vi "Controls Loop.vi"(8 "error in":errorcluster, 10 "Controls[]":refnum<vi>[](array[refnum]), 11 "Material-Scheme in":refnum<class "Material-Scheme.lvclass">) -> (0 "error out":errorcluster)   [LabVIEW 2021, in "TSC Material Theme.lvlib" / "Material-Scheme.lvclass"]
doc: "loop through all the controls on a panel in order to change the appearance\n\n<b>Code Developed By:</b>\nTechnology Service Corporation\nwww.tsc.com/atcs\n\nDeveloper:\nDaniel Coons"
uses:
  Material-Scheme.lvclass
  Material-Scheme.lvclass/Material-Scheme.ctl
  <vilib>/Utility/miscctls.llb/LVRowAndColumnTypeDef.ctl
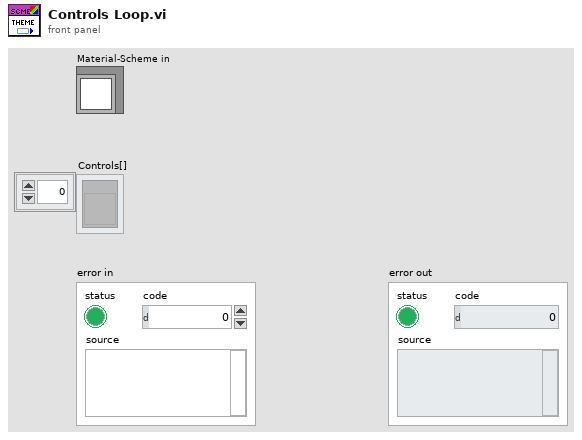
[diagram p1: front panel]
types:
  T1 = typedef "LVRowAndColumnTypeDef.ctl" = cluster{"Row":i32, "Column":i32}
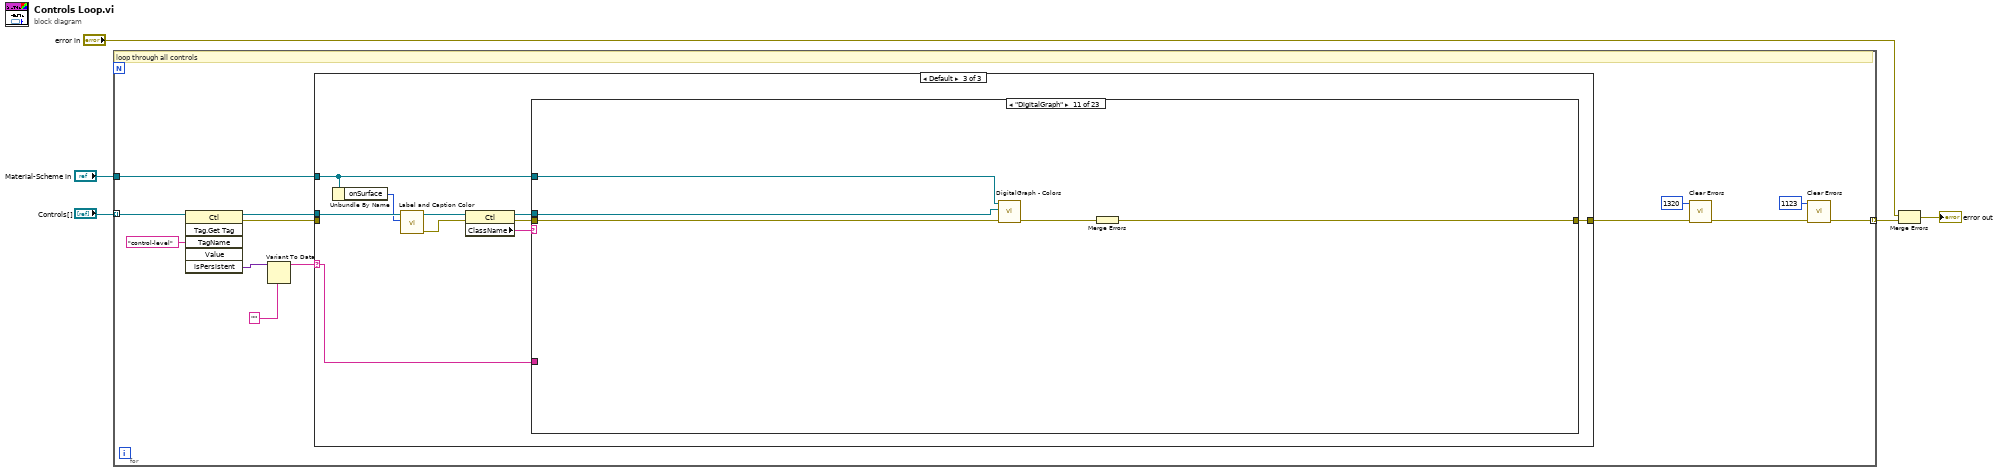
[diagram p0: block diagram]
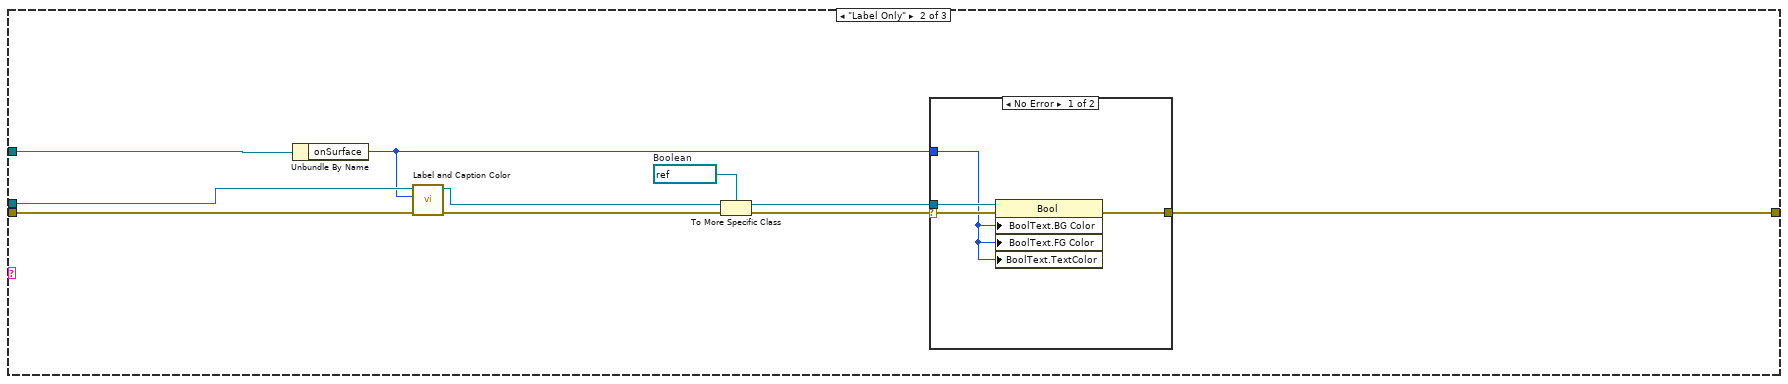
[diagram p3: hidden frame]
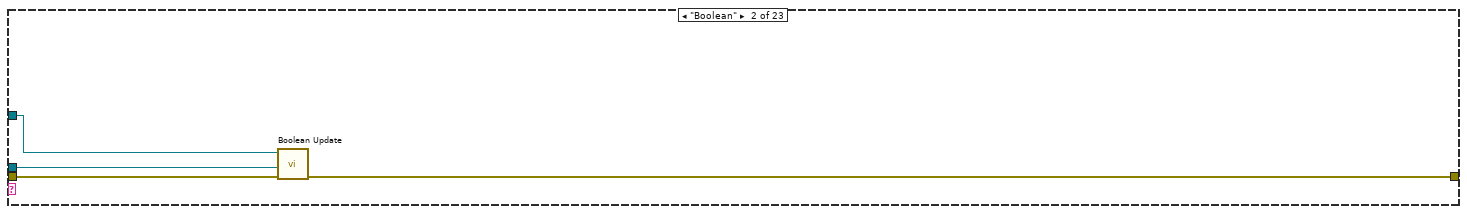
[diagram p6: hidden frame]
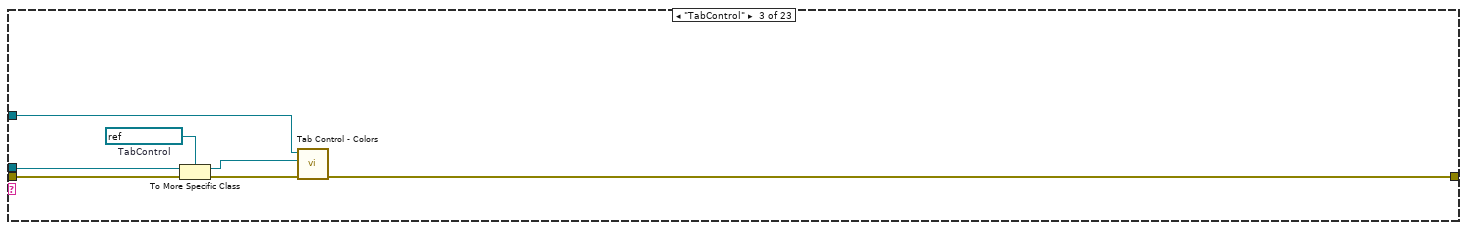
[diagram p7: hidden frame]
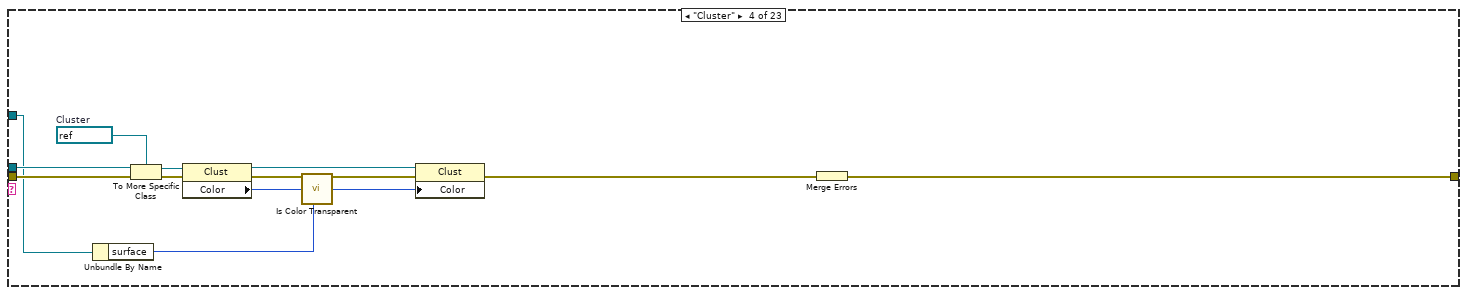
[diagram p8: hidden frame]
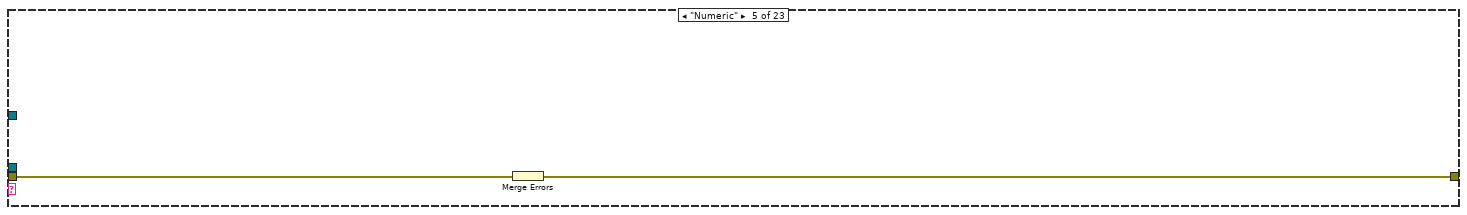
[diagram p9: hidden frame]
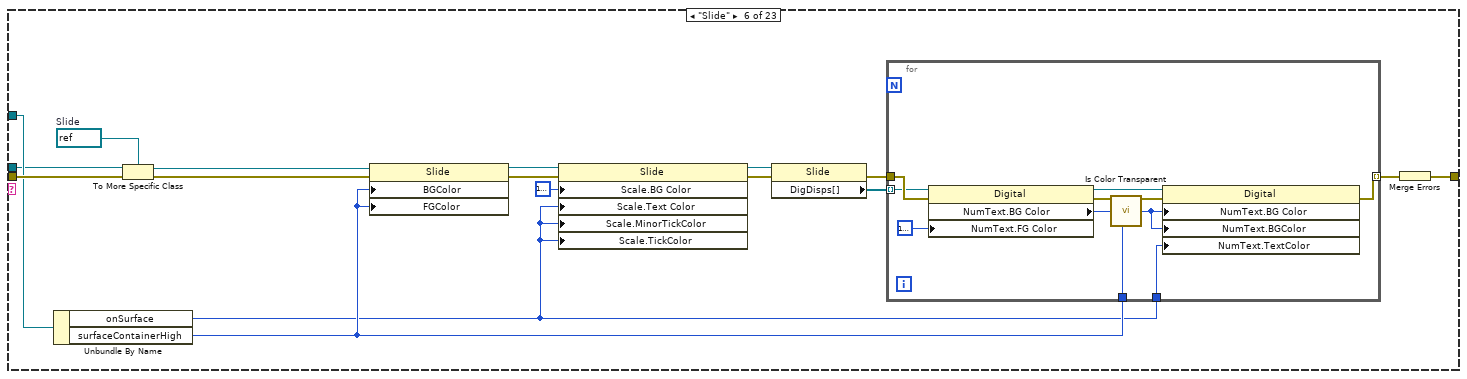
[diagram p10: hidden frame]
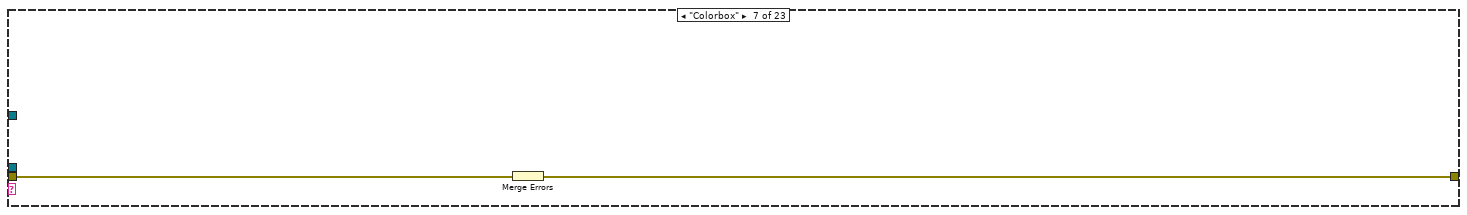
[diagram p11: hidden frame]
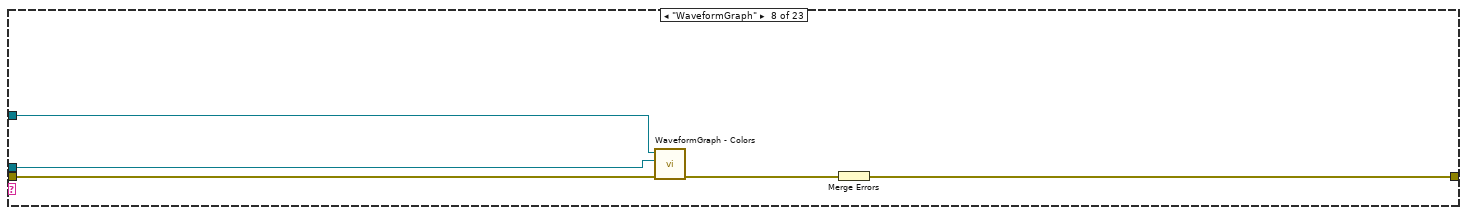
[diagram p12: hidden frame]
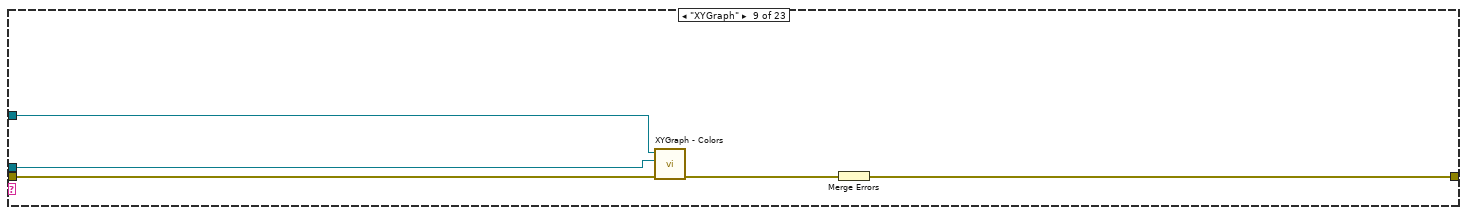
[diagram p13: hidden frame]
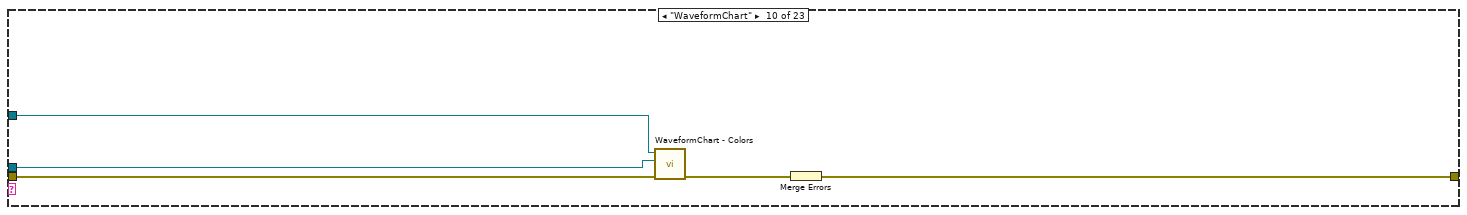
[diagram p14: hidden frame]
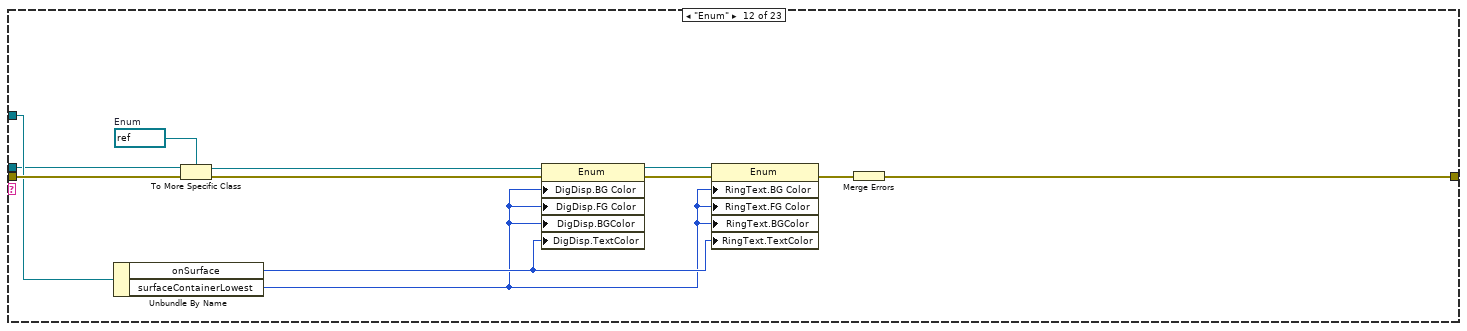
[diagram p15: hidden frame]
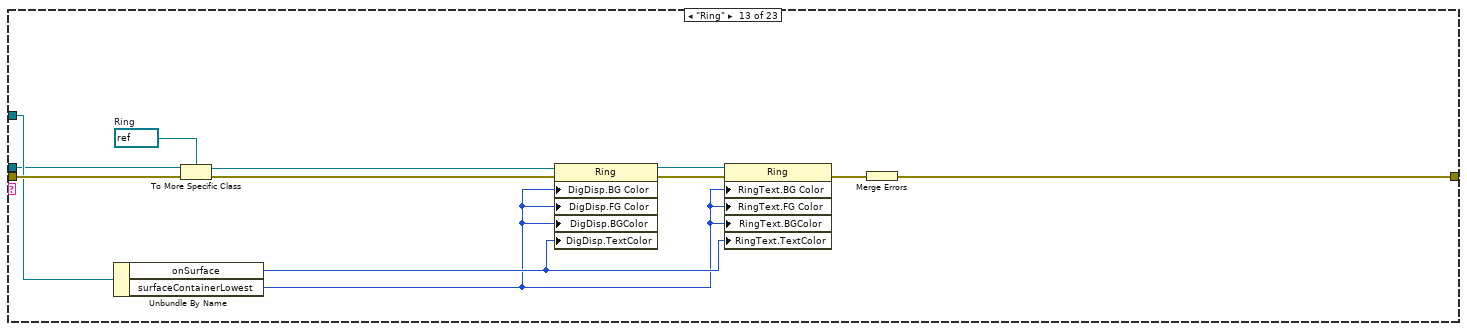
[diagram p16: hidden frame]
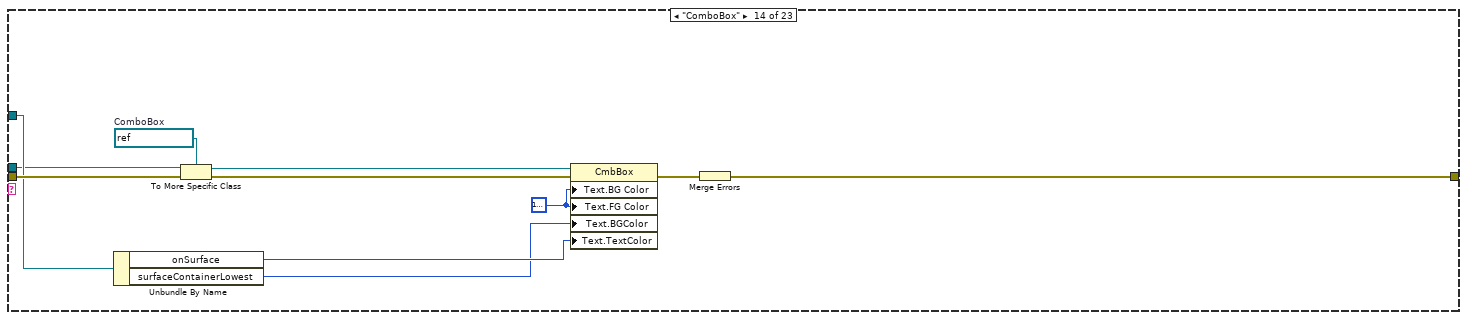
[diagram p17: hidden frame]
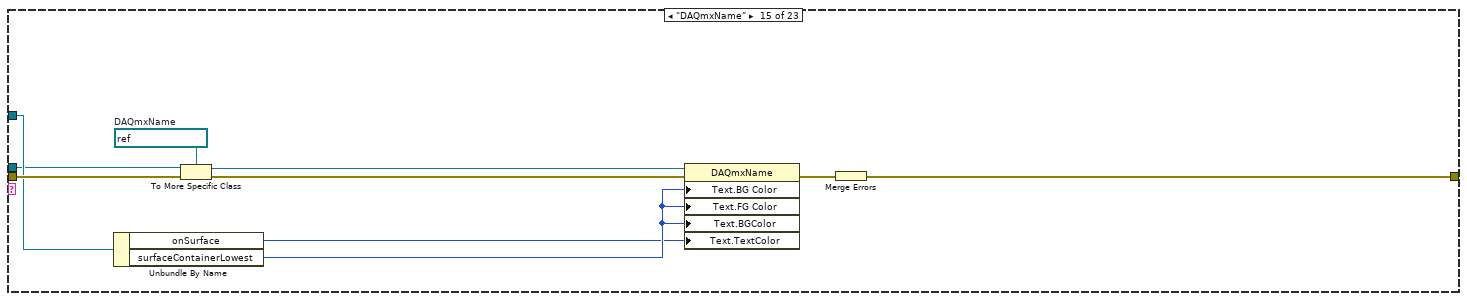
[diagram p18: hidden frame]
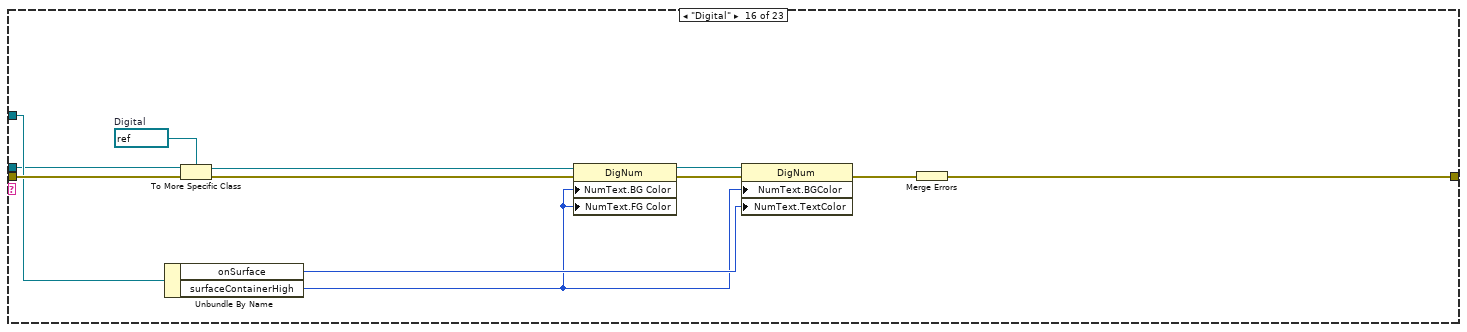
[diagram p19: hidden frame]
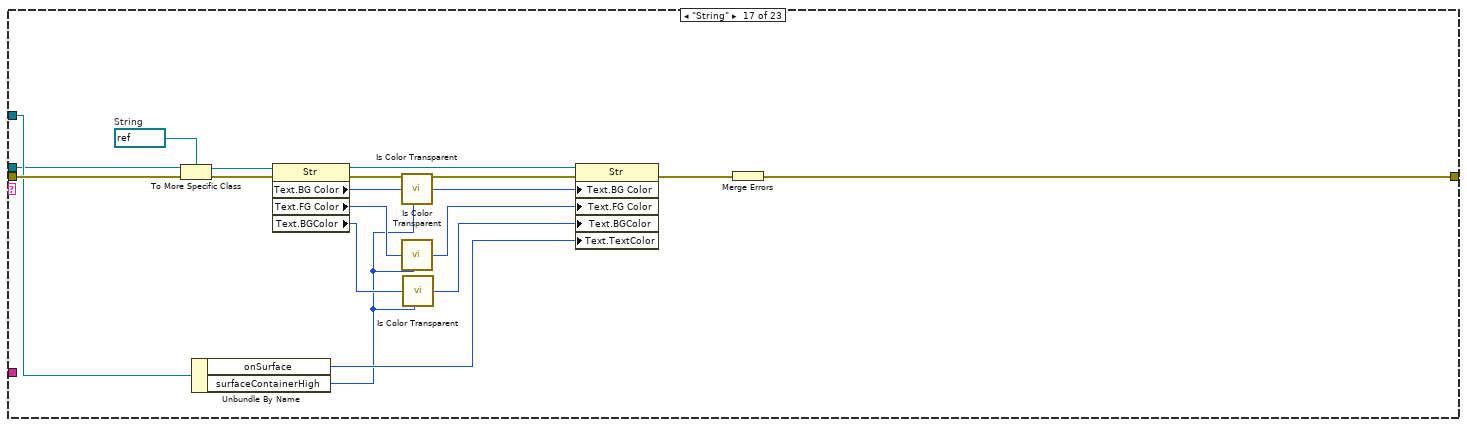
[diagram p20: hidden frame]
diagram:
  n1 = for {
    tunnel: "Controls[]" -> [w15] mode=indexing
    tunnel: "Material-Scheme in" -> [w18]
    tunnel: [w7] -> w3 mode=indexing
    # "loop through all controls"
    n2 = invoke class="Ctl" method="Tag.Get Tag"(reference=w15, "TagName"="control-level" ("Tag Name")) -> (reference out=w14:refnum<vi>, error out=w10:errorcluster, "isPersistent"=w13:variant)  [unwired: 4 in, 3 out]
    n3 = Variant To Data(type="", Variant=w13) -> (data=w11:string)  [unwired: 1 in, 1 out]
    n4 = case shown="Default" w11 {
      selector: w11 -> [_ _ w39]
      tunnel: w14 -> [_ w22 w38]
      tunnel: w18 -> [_ w28 w35]
      tunnel: [w19 w24 w40] -> w17
      tunnel: w10 -> [w19 w29 _]
      frame "N/A", "no change", "no-change" {
      }
      frame "Label Only" {
        w27 = refnum<vi> refnum  # Boolean
        n5 = Unbundle By Name(w28) -> ("onSurface"=w20:u32)
        n6 = call "Label and Caption Color.vi"("error in"=w29, "Text Color"=w20, "ctrl ref in"=w22) -> ("error out"=w23:errorcluster, "ctrl ref out"=w21:refnum<vi>)  [unwired: 7 in]
        n7 = To More Specific Class(target class=w27, reference=w21, error in=w23) -> (specific class reference=w26:refnum<vi>, error out=w25:errorcluster)
        n8 = case shown="No Error" w25 {
          selector: w25 -> [w32 _]
          tunnel: w26 -> [w33 _]
          tunnel: w20 -> [w31 _]
          tunnel: [w30 _] -> w24
          frame No Error {
            n9 = property class="Bool"(reference=w33, error in=w32, "BoolText.BG Color"=w31, "BoolText.FG Color"=w31, "BoolText.TextColor"=w31) -> (error out=w30:errorcluster)  [unwired: 1 out]
          }
          frame Error {
          }
        }
      }
      frame Default {
        n10 = Unbundle By Name(w35) -> ("onSurface"=w34:u32)
        n11 = call "Label and Caption Color.vi"("Text Color"=w34, "ctrl ref in"=w38) -> ("error out"=w36:errorcluster, "ctrl ref out"=w37:refnum<vi>)  [unwired: 8 in]
        n12 = property class="Ctl"(reference=w37, error in=w36) -> (reference out=w42:refnum<vi>, error out=w41:errorcluster, "ClassName"=w43:string)
        n13 = case shown="\"DigitalGraph\"" w43 {
          tunnel: w42 -> [_ w45 w51 w67 _ w85 _ w101 w106 w111 w116 w127 w139 w150 w160 w172 w189 w198 w208 w219 w241 w268 w288]
          tunnel: w41 -> [w44 w48 w52 w66 w70 w87 w99 w104 w109 w114 w119 w131 w143 w154 w164 w176 w194 w199 w207 w220 w242 w269 w289]
          tunnel: w35 -> [_ w47 w54 w63 _ w86 _ w102 w107 w112 w117 w129 w141 w152 w162 w174 w191 _ w204 w212 w235 w257 w275]
          tunnel: [w44 w46 w55 w64 w69 w73 w98 w103 w108 w113 w118 w130 w142 w153 w163 w175 w193 w196 w205 w214 w224 w259 w277] -> w40
          tunnel: w39 -> [_ _ _ _ _ _ _ _ _ _ _ _ _ _ _ _ _ _ _ w211 w236 w256 w274]
          frame Default {
          }
          frame "Boolean" {
            n14 = call "Boolean Update.vi"("error in (no error)"=w48, "Control in"=w45, "Material-Scheme.lvclass"=w47) -> ("error out"=w46:errorcluster)  [unwired: 8 in]
          }
          frame "TabControl" {
            w53 = refnum<vi> refnum  # TabControl
            n15 = To More Specific Class(target class=w53, reference=w51, error in=w52) -> (specific class reference=w50:refnum<vi>, error out=w49:errorcluster)
            n16 = call "Tab Control - Colors.vi"("error in (no error)"=w49, "ctrl ref in"=w50, "Material-Scheme in"=w54) -> ("error out"=w55:errorcluster)  [unwired: 8 in]
          }
          frame "Cluster" {
            w68 = refnum<vi> refnum  # Cluster
            n17 = Unbundle By Name(w63) -> ("surface"=w57:u32)
            n18 = To More Specific Class(target class=w68, reference=w67, error in=w66) -> (specific class reference=w61:refnum<vi>, error out=w65:errorcluster)
            n19 = property class="Clust"(reference=w61, error in=w65) -> (reference out=w60:refnum<vi>, error out=w62:errorcluster, "Color"=w58:u32)
            n20 = call "Is Color Transparent.vi"("original color"=w58, "desired color"=w57) -> ("updated color"=w59:u32)  [unwired: 3 in]
            n21 = property class="Clust"(reference=w60, error in=w62, "Color"=w59) -> (error out=w56:errorcluster)  [unwired: 1 out]
            n22 = Merge Errors(w56) -> (w64:errorcluster)
          }
          frame "Numeric" {
            n23 = Merge Errors(w70) -> (w69:errorcluster)
          }
          frame "Slide" {
            w84 = refnum<vi> refnum  # Slide
            n24 = Unbundle By Name(w86) -> ("onSurface"=w75:u32, "surfaceContainerHigh"=w76:u32)
            n25 = To More Specific Class(target class=w84, reference=w85, error in=w87) -> (specific class reference=w71:refnum<vi>, error out=w72:errorcluster)
            n26 = property class="Slide"(reference=w71, error in=w72, "BGColor"=w76, "FGColor"=w76) -> (reference out=w82:refnum<vi>, error out=w83:errorcluster)
            n27 = property class="Slide"(reference=w82, error in=w83, "Scale.BG Color"=u32 16777216 ("Scale.Marker Colors:BG Color"), "Scale.Text Color"=w75, "Scale.MinorTickColor"=w75, "Scale.TickColor"=w75) -> (reference out=w79:refnum<vi>, error out=w80:errorcluster)
            n28 = property class="Slide"(reference=w79, error in=w80) -> (error out=w78:errorcluster, "DigDisps[]"=w77:refnum<vi>[])  [unwired: 1 out]
            n29 = for {
              tunnel: w78 -> [w97]
              tunnel: w77 -> [w96] mode=indexing
              tunnel: w76 -> [w92]
              tunnel: w75 -> [w89]
              tunnel: [w88] -> w74 mode=indexing
              n30 = property class="Digital"(reference=w96, error in=w97, "NumText.FG Color"=u32 16777216 ("Numeric Text.Colors:FG Color")) -> (reference out=w94:refnum<vi>, error out=w93:errorcluster, "NumText.BG Color"=w91:u32)
              n31 = call "Is Color Transparent.vi"("original color"=w91, "desired color"=w92) -> ("updated color"=w90:u32)  [unwired: 3 in]
              n32 = property class="Digital"(reference=w94, error in=w93, "NumText.BG Color"=w90, "NumText.BGColor"=w90, "NumText.TextColor"=w89) -> (error out=w88:errorcluster)  [unwired: 1 out]
            }
            n33 = Merge Errors(w74) -> (w73:errorcluster)
          }
          frame "Colorbox" {
            n34 = Merge Errors(w99) -> (w98:errorcluster)
          }
          frame "WaveformGraph" {
            n35 = call "WaveformGraph - Colors.vi"("error in"=w104, "Ctl Refnum"=w101, "Material-Scheme in"=w102) -> ("error out"=w100:errorcluster)  [unwired: 8 in]
            n36 = Merge Errors(w100) -> (w103:errorcluster)
          }
          frame "XYGraph" {
            n37 = call "XYGraph - Colors.vi"("error in"=w109, "Ctl Refnum"=w106, "Material-Scheme in"=w107) -> ("error out"=w105:errorcluster)  [unwired: 8 in]
            n38 = Merge Errors(w105) -> (w108:errorcluster)
          }
          frame "WaveformChart" {
            n39 = call "WaveformChart - Colors.vi"("error in (no error)"=w114, "Ctl Refnum"=w111, "Material-Scheme in"=w112) -> ("error out"=w110:errorcluster)  [unwired: 8 in]
            n40 = Merge Errors(w110) -> (w113:errorcluster)
          }
          frame "DigitalGraph" {
            n41 = call "DigitalGraph - Colors.vi"("error in (no error)"=w119, "Ctl Refnum"=w116, "Material-Scheme in"=w117) -> ("error out"=w115:errorcluster)  [unwired: 8 in]
            n42 = Merge Errors(w115) -> (w118:errorcluster)
          }
          frame "Enum" {
            w125 = refnum<vi> refnum  # Enum
            n43 = Unbundle By Name(w129) -> ("onSurface"=w123:u32, "surfaceContainerLowest"=w121:u32)
            n44 = To More Specific Class(target class=w125, reference=w127, error in=w131) -> (specific class reference=w126:refnum<vi>, error out=w128:errorcluster)
            n45 = property class="Enum"(reference=w126, error in=w128, "DigDisp.BG Color"=w121, "DigDisp.FG Color"=w121, "DigDisp.BGColor"=w121, "DigDisp.TextColor"=w123) -> (reference out=w120:refnum<vi>, error out=w124:errorcluster)
            n46 = property class="Enum"(reference=w120, error in=w124, "RingText.BG Color"=w121, "RingText.FG Color"=w121, "RingText.BGColor"=w121, "RingText.TextColor"=w123) -> (error out=w122:errorcluster)  [unwired: 1 out]
            n47 = Merge Errors(w122) -> (w130:errorcluster)
          }
          frame "Ring" {
            w137 = refnum<vi> refnum  # Ring
            n48 = Unbundle By Name(w141) -> ("onSurface"=w135:u32, "surfaceContainerLowest"=w133:u32)
            n49 = To More Specific Class(target class=w137, reference=w139, error in=w143) -> (specific class reference=w138:refnum<vi>, error out=w140:errorcluster)
            n50 = property class="Ring"(reference=w138, error in=w140, "DigDisp.BG Color"=w133, "DigDisp.FG Color"=w133, "DigDisp.BGColor"=w133, "DigDisp.TextColor"=w135) -> (reference out=w132:refnum<vi>, error out=w136:errorcluster)
            n51 = property class="Ring"(reference=w132, error in=w136, "RingText.BG Color"=w133, "RingText.FG Color"=w133, "RingText.BGColor"=w133, "RingText.TextColor"=w135) -> (error out=w134:errorcluster)  [unwired: 1 out]
            n52 = Merge Errors(w134) -> (w142:errorcluster)
          }
          frame "ComboBox" {
            w144 = u32 16777216 ("Text.Colors:FG Color")
            w148 = refnum<vi> refnum  # ComboBox
            n53 = Unbundle By Name(w152) -> ("onSurface"=w146:u32, "surfaceContainerLowest"=w145:u32)
            n54 = To More Specific Class(target class=w148, reference=w150, error in=w154) -> (specific class reference=w149:refnum<vi>, error out=w151:errorcluster)
            n55 = property class="CmbBox"(reference=w149, error in=w151, "Text.BG Color"=w144, "Text.FG Color"=w144, "Text.BGColor"=w145, "Text.TextColor"=w146) -> (error out=w147:errorcluster)  [unwired: 1 out]
            n56 = Merge Errors(w147) -> (w153:errorcluster)
          }
          frame "DAQmxName" {
            w158 = refnum<vi> refnum  # DAQmxName
            n57 = Unbundle By Name(w162) -> ("onSurface"=w155:u32, "surfaceContainerLowest"=w156:u32)
            n58 = To More Specific Class(target class=w158, reference=w160, error in=w164) -> (specific class reference=w159:refnum<vi>, error out=w161:errorcluster)
            n59 = property class="DAQmxName"(reference=w159, error in=w161, "Text.BG Color"=w156, "Text.FG Color"=w156, "Text.BGColor"=w156, "Text.TextColor"=w155) -> (error out=w157:errorcluster)  [unwired: 1 out]
            n60 = Merge Errors(w157) -> (w163:errorcluster)
          }
          frame "Digital" {
            w170 = refnum<vi> refnum  # Digital
            n61 = Unbundle By Name(w174) -> ("onSurface"=w166:u32, "surfaceContainerHigh"=w165:u32)
            n62 = To More Specific Class(target class=w170, reference=w172, error in=w176) -> (specific class reference=w171:refnum<vi>, error out=w173:errorcluster)
            n63 = property class="DigNum"(reference=w171, error in=w173, "NumText.BG Color"=w165, "NumText.FG Color"=w165) -> (reference out=w167:refnum<vi>, error out=w169:errorcluster)
            n64 = property class="DigNum"(reference=w167, error in=w169, "NumText.BGColor"=w165, "NumText.TextColor"=w166) -> (error out=w168:errorcluster)  [unwired: 1 out]
            n65 = Merge Errors(w168) -> (w175:errorcluster)
          }
          frame "String" {
            w188 = refnum<vi> refnum  # String
            n66 = To More Specific Class(target class=w188, reference=w189, error in=w194) -> (specific class reference=w185:refnum<vi>, error out=w190:errorcluster)
            n67 = Unbundle By Name(w191) -> ("onSurface"=w187:u32, "surfaceContainerHigh"=w180:u32)
            n68 = property class="Str"(reference=w185, error in=w190) -> (reference out=w184:refnum<vi>, error out=w186:errorcluster, "Text.BG Color"=w183:u32, "Text.FG Color"=w182:u32, "Text.BGColor"=w181:u32)
            n69 = call "Is Color Transparent.vi"("original color"=w183, "desired color"=w180) -> ("updated color"=w177:u32)  [unwired: 3 in]
            n70 = call "Is Color Transparent.vi"("original color"=w182, "desired color"=w180) -> ("updated color"=w178:u32)  [unwired: 3 in]
            n71 = call "Is Color Transparent.vi"("original color"=w181, "desired color"=w180) -> ("updated color"=w179:u32)  [unwired: 3 in]
            n72 = property class="Str"(reference=w184, error in=w186, "Text.BG Color"=w177, "Text.FG Color"=w178, "Text.BGColor"=w179, "Text.TextColor"=w187) -> (error out=w192:errorcluster)  [unwired: 1 out]
            n73 = Merge Errors(w192) -> (w193:errorcluster)
          }
          frame "Array" {
            w197 = refnum<vi> refnum  # Array
            n74 = To More Specific Class(target class=w197, reference=w198, error in=w199) -> (error out=w195:errorcluster)  [unwired: 1 out]
            n75 = Merge Errors(w195) -> (w196:errorcluster)
          }
          frame "Path" {
            w209 = refnum<vi> refnum  # Path
            n76 = Unbundle By Name(w204) -> ("surfaceContainerHigh"=w202:u32, "onSurface"=w200:u32)
            n77 = To More Specific Class(target class=w209, reference=w208, error in=w207) -> (specific class reference=w203:refnum<vi>, error out=w206:errorcluster)
            n78 = property class="Path"(reference=w203, error in=w206, "Text.BG Color"=w202, "Text.FG Color"=w202, "Text.FontColor"=w200, "Text.BGColor"=w202, "Text.TextColor"=w200) -> (error out=w201:errorcluster)  [unwired: 1 out]
            n79 = Merge Errors(w201) -> (w205:errorcluster)
          }
          frame "ListBox" {
            w221 = refnum<vi> refnum  # ListBox
            n80 = To More Specific Class(target class=w221, reference=w219, error in=w220) -> (specific class reference=w217:refnum<vi>, error out=w218:errorcluster)
            n81 = call "Color Grabber.vi"("control-level"=w211, "Material-Scheme in"=w212) -> ("colorContainer"=w210:u32)  [unwired: 3 in, 6 out]
            n82 = Unbundle By Name(w212) -> ("surfaceContainerLowest"=w215:u32, "onSurface"=w213:u32)
            n83 = property class="LstBox"(reference=w217, error in=w218, "Active Row"=-2 ("Active Row:Active Row Number"), "CellBG"=w215, "CellFontColor"=w213, "SelColor"=w210) -> (error out=w214:errorcluster)  [unwired: 1 out]
          }
          frame "TreeControl" {
            w238 = -2 ("Active Row:Active Row Number")
            w243 = refnum<vi> refnum  # TreeControl
            n84 = Unbundle By Name(w235) -> ("surfaceContainerLowest"=w237:u32, "onSurface"=w223:u32)
            n85 = To More Specific Class(target class=w243, reference=w241, error in=w242) -> (specific class reference=w239:refnum<vi>, error out=w240:errorcluster)
            n86 = call "Color Grabber.vi"("control-level"=w236, "Material-Scheme in"=w235) -> ("onColor"=w225:u32, "color"=w226:u32, "colorContainer"=w222:u32)  [unwired: 3 in, 4 out]
            n87 = property class="Tree"(reference=w239, error in=w240, "Active Item Row Number"=w238, "ActiveColNum"=w238, "CellBG"=w237, "CellFontColor"=w223, "SelColor"=w222) -> (reference out=w233:refnum<vi>, error out=w234:errorcluster)
            n88 = property class="Tree"(reference=w233, error in=w234, "Active Item Row Number"=-1 ("Active Row:Active Row Number"), "ActiveColNum"=-2 ("Active Row:Active Row Number"), "CellBG"=w226, "CellFontColor"=w225) -> (reference out=w229:refnum<vi>, error out=w230:errorcluster)
            n89 = property class="Tree"(reference=w229, error in=w230, "Active Item Row Number"=-2 ("Active Row:Active Row Number"), "ActiveColNum"=-1 ("Active Row:Active Row Number"), "CellBG"=w226, "CellFontColor"=w225) -> (error out=w224:errorcluster)  [unwired: 1 out]
          }
          frame "MulticolumnListbox" {
            w270 = refnum<vi> refnum  # MulticolumnListbox
            # "check for variations of dark\nand remove horizontal lines"
            # "header"
            n90 = To More Specific Class(target class=w270, reference=w268, error in=w269) -> (specific class reference=w266:refnum<vi>, error out=w267:errorcluster)
            n91 = Unbundle By Name(w257) -> ("surfaceContainerLowest"=w264:u32, "onSurface"=w258:u32)
            n92 = call "Color Grabber.vi"("control-level"=w256, "Material-Scheme in"=w257) -> ("onColor"=w251:u32, "color"=w252:u32, "colorContainer"=w248:u32)  [unwired: 3 in, 4 out]
            n93 = property class="Material-Scheme"(reference=w257) -> ("data member access:name"=w260:string)  [unwired: 1 in, 2 out]
            n94 = property class="MCListbox"(reference=w266, error in=w267, "ActiveCell"=T1 {"Row"=-2, "Column"=-2} ("Active Cell:Active Cell"), "CellBG"=w264, "CellFontColor"=w258) -> (reference out=w262:refnum<vi>, error out=w263:errorcluster)
            n95 = To Lower Case(string=w260) -> (all lower case string=w247:string)
            n96 = property class="MCListbox"(reference=w262, error in=w263, "ActiveCell"=T1 {"Row"=-1, "Column"=-2} ("Active Cell:Active Cell"), "CellBG"=w252, "CellFontColor"=w251, "SelColor"=w248) -> (reference out=w254:refnum<vi>, error out=w255:errorcluster)
            n97 = property class="MCListbox"(reference=w254, error in=w255, "ActiveCell"=T1 {"Row"=-2, "Column"=-1} ("Active Cell:Active Cell"), "CellBG"=w252, "CellFontColor"=w251, "SelColor"=w248) -> (reference out=w249:refnum<vi>, error out=w250:errorcluster)
            n98 = Match Pattern(string=w247, regular expression="dark" ("y")) -> (offset past match=w245:i32)  [unwired: 1 in, 3 out]
            n99 = Less Than 0?(x=w245) -> (x < 0?=w244:bool)
            n100 = property class="MCListbox"(reference=w249, error in=w250, "Horizontal Lines Visible"=w244) -> (error out=w259:errorcluster)  [unwired: 1 out]
          }
          frame "Table" {
            w290 = refnum<vi> refnum  # Table
            n101 = To More Specific Class(target class=w290, reference=w288, error in=w289) -> (specific class reference=w286:refnum<vi>, error out=w287:errorcluster)
            n102 = Unbundle By Name(w275) -> ("surfaceContainerLowest"=w284:u32, "onSurface"=w280:u32)
            n103 = call "Color Grabber.vi"("control-level"=w274, "Material-Scheme in"=w275) -> ("onColor"=w272:u32, "color"=w273:u32, "colorContainer"=w271:u32)  [unwired: 3 in, 4 out]
            n104 = property class="Tbl"(reference=w286, error in=w287, "Active Cell"=T1 {"Row"=-2, "Column"=-2} ("Active Cell:Active Cell"), "Cell BG Color"=w284, "CellFontColor"=w280) -> (reference out=w282:refnum<vi>, error out=w283:errorcluster)
            n105 = property class="Tbl"(reference=w282, error in=w283, "Active Cell"=T1 {"Row"=-1, "Column"=-2} ("Active Cell:Active Cell"), "Cell BG Color"=w273, "CellFontColor"=w272, "Selection Color"=w271) -> (reference out=w278:refnum<vi>, error out=w279:errorcluster)
            n106 = property class="Tbl"(reference=w278, error in=w279, "Active Cell"=T1 {"Row"=-2, "Column"=-1} ("Active Cell:Active Cell"), "Cell BG Color"=w273, "CellFontColor"=w272, "Selection Color"=w271) -> (error out=w277:errorcluster)  [unwired: 1 out]
          }
        }
      }
    }
    n107 = call <vilib>:"Clear Errors.vi"("error in (no error)"=w17, "specific error code to clear (0: all)"=1320) -> ("error out"=w9:errorcluster)  [unwired: 4 in, 1 out]
    n108 = call <vilib>:"Clear Errors.vi"("error in (no error)"=w9, "specific error code to clear (0: all)"=1123) -> ("error out"=w7:errorcluster)  [unwired: 4 in, 1 out]
  }
  n109 = Merge Errors("error in", w3) -> (→"error out":errorcluster)
